vi "Update Parameters Configuration File MD5 Error.vi"(8 "error in":errorcluster, 11 "configuration files ref":T1 format="%.0x") -> (0 "error out":errorcluster, 3 "configuration files ref out":T1 format="%.0x")   [LabVIEW 2020, in "Ballard ARINC 429 Scripting.lvlib"]
uses:
  Ballard ARINC 429 Scripting.lvlib
  <vilib>/NI VeriStand/Custom Device API/Custom Device Item Ref.ctl
  <vilib>/NI VeriStand/Custom Device API/Custom Device API.lvlib
  Constants.vi
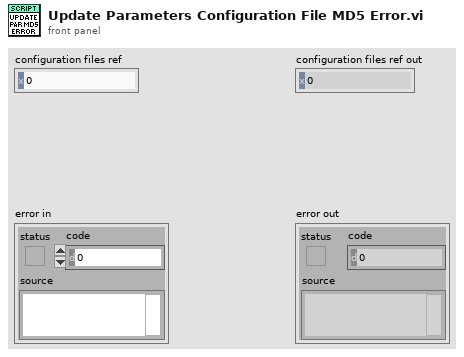
[diagram p1: front panel]
types:
  T1 = typedef "Custom Device API.lvlib/Custom Device Item Ref.ctl" = u64
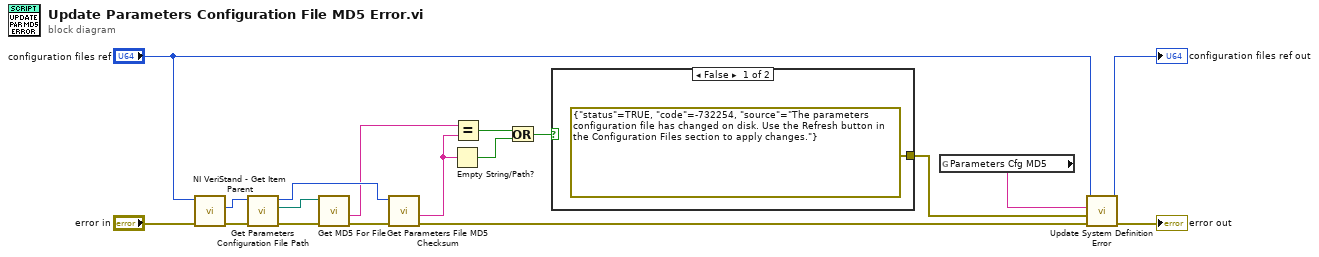
[diagram p0: block diagram]
diagram:
  n1 = call <vilib>:"NI VeriStand - Get Item Parent.vi"("error in (no error)"="error in", "Item Ref in"="configuration files ref") -> ("error out"=w9:errorcluster, "Parent Ref"=w11:T1)  [unwired: 6 in, 2 out]
  n2 = call "Get Parameters Configuration File Path.vi"("error in"=w9, "custom device ref"=w11) -> ("error out"=w6:errorcluster, "path"=w5:path, "custom device ref out"=w4:T1)  [unwired: 6 in, 1 out]
  n3 = call "Get MD5 For File.vi"("error in"=w6, "path"=w5) -> ("error out"=w2:errorcluster, "MD5"=w3:string)  [unwired: 8 in]
  n4 = call "Get Parameters File MD5 Checksum.vi"("error in"=w2, "custom device ref"=w4) -> ("error out"=w7:errorcluster, "MD5"=w12:string)  [unwired: 7 in, 1 out]
  n5 = Empty String/Path?(string/path=w12) -> (empty?=w15:bool)
  n6 = Equal?(x=w3, y=w12) -> (x = y?=w14:bool)
  n7 = Or(x=w14, y=w15) -> (x .or. y?=w13:bool)
  n8 = case shown="False" w13 {
    tunnel: [errorcluster {"status"=TRUE, "code"=-732254, "source"="The parameters configuration file has changed on disk. Use the Refresh button in the Configuration Files section to apply changes."} ("New Error") _] -> w16
    frame False {
    }
    frame True {
      # "No error if MD5s are equal or one doesn't exist."
    }
  }
  n9 = global read "Constants.vi" "Parameters Cfg MD5"() -> (w1:string)
  n10 = call "Update System Definition Error.vi"("error to report"=w7, "error in"=w16, "error key"=w1, "Configuration files Ref"="configuration files ref") -> ("error out"=→"error out":errorcluster, "Configuration files Ref out"=→"configuration files ref out":T1)  [unwired: 6 in]
